vi "Robot Global Data.vi"() -> ()   [LabVIEW 2019]
doc: "This global VI can contain as many global variables as you need. To create a global variable, place a control on the panel, give it a good name. To read or write to it from a VI, drag the icon to the diagram of that VI. You can also drag from the project. Click on the node to change which global you access. You shouldn't have multiple locations writing to a global or it will cause a race-condition."
uses:
  <vilib>/Rock Robotics/WPI/Camera/WPI_CameraImageSize.ctl
  <vilib>/Rock Robotics/WPI/DriverStation/WPI_DriverStationRobotMode2.ctl
panel:
  in  "Transfer Duration":dbl=0.5
  in  "Transfer Set Point":dbl=0.5
  in  "Shooter Duration":dbl=0.5
  in  "Shooter Set Point":dbl=0.5
  in  "Intake Duration":dbl=0.5
  in  "Intake Set Point":dbl=0.5
  in  "AimDeadband":dbl min=0.0 max=10.0 step=0.25
  in  "SteeringK":dbl(slide)=0.025362318840579712 min=0.0 max=0.25 step=0.01 scale=0.0..0.25
  in  "MinSteerCommand":dbl(slide)=0.2717391304347826 min=0.0 max=0.5 step=0.05 scale=0.0..0.5
  in  "Limelight Goal Area":dbl(slide)=14.872262773722628 min=0.1 max=25.0 step=0.25 scale=0.0..25.0
  in  "DriveK":dbl(slide)=0.26277372262773724 min=0.0 max=1.0 step=0.05 scale=0.0..1.0
  in  "MaxDrive":dbl(slide)=0.6824817518248175 min=0.0 max=1.0 step=0.01 scale=0.0..1.0
  in  "DriveScale":dbl(slide)=0.7556179775280899 min=0.25 max=1.0 step=0.1 scale=0.25..1.0
  in  "Steering Scale":dbl(slide)=0.6418539325842696 min=0.25 max=1.0 step=0.1 scale=0.25..1.0
  in  "MaxSpeedSlow":dbl=0.4
  in  "SlowRate":dbl=1.0
  in  "MaxTurnSlow":dbl=0.55
  in  "MaxTurnRateSlow":dbl=20.0
  in  "SlowModeSettings":i32=2
  in  "Cheezy Drive Mode":u32=2
  out "tv - valid target":dbl
  out "Op. Button 7":bool
  out "Op. Button 6":bool
  out "Op. Button 5":bool
  out "Op. Button 4":bool
  out "Op. Button 3":bool
  out "Op. Button 2":bool
  out "Op. Button 1":bool
  out "Op. Button 0":bool
  in  "y axis":dbl
  in  "x axis":dbl
  out "Button 7":bool
  out "Button 6":bool
  out "Button 5":bool
  out "Button 4":bool
  out "Button 3":bool
  out "Button 2":bool
  out "Button 1":bool
  out "Button 0":bool
  out "tx - offsetAngle H":dbl
  out "ty - offsetAngle V":dbl
  out "ta - area":dbl
  out "ts - skew":dbl
  in  "Right Pivot":bool
  in  "Left Pivot":bool
  in  "SlowMode":u32=2
  in  "Quickturn":bool
  in  "Select Mode":dbl
  in  "Speed":dbl
  in  "Turn":dbl
  in  "Robot Mode":T1
  in  "image size":T2=enum."320x240"
  in  "Enable Vision":bool
  # "Cheezy Drive Settings"
  # "Drive Settings"
  # "Limelight Variables"
  # "Limelight Drive Variables"
  # "Driver Joystick Variables"
  # "Operator Joystick Variables"
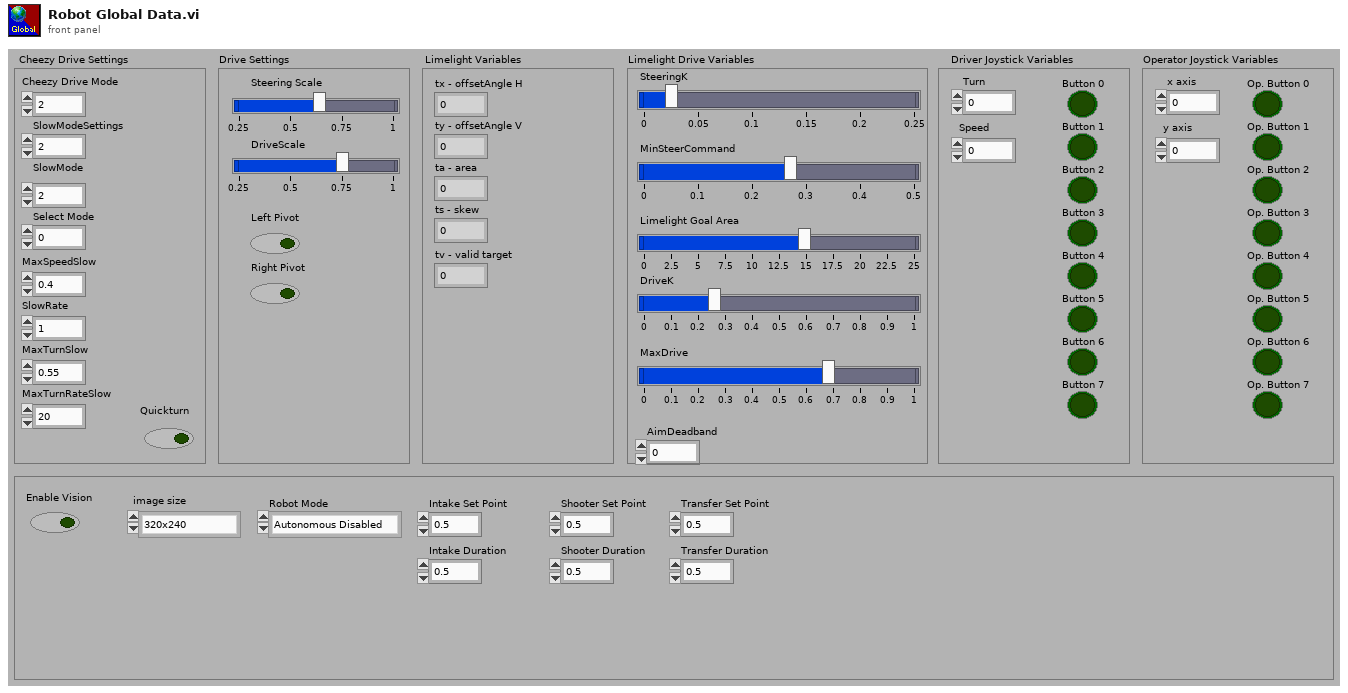
[diagram p1: front panel]
types:
  T1 = typedef "WPI_DriverStationRobotMode2.ctl" = enum16{"Autonomous Disabled", "Autonomous Enabled", "Teleop Disabled", "Teleop Enabled", "Disconnected", "Finish", "Test Disabled", "Test Enabled", "Emergency Stopped"}
  T2 = typedef "WPI_CameraImageSize.ctl" = enum16{"640x480", "320x240", "160x120", "Custom"}
diagram:
